vi "rscmwLS-lv2010_LTE_Signaling_example-1.0.0.vi"() -> ()   [LabVIEW 2010]
uses:
  <vilib>/Utility/error.llb/DialogType.ctl
panel:
  out "Error during execution?":bool
  out "State Indicator":T1(ring)
  out "RSRQ range":string
  out "RSRP range":string
  out "RSRQ":i32
  out "RSRP":i32
  out "error out":errorcluster
  in  "Set Type (Alternative Pattern)":i32(ring)=4 items=["Minimum Power", "Maximum Power", "Constant", "Single Pattern", "Closed Loop Target Power", "Different Pattern", "Continuous Pattern", "Alternative Pattern", "Relative Power Control"]
  in  "PUSCH Closed Loop Target Power (-20.0)":dbl=-20.0 caption="Power (-20.0)" format="%^.3e"
  in  "PUSCH Open Loop Nominal Power (-20.0)":dbl=-20.0 caption="Open Loop Nominal Power (-20.0)" format="%^.3e"
  in  "RS EPRE (-85.0)":dbl=-85.0 format="%^.3e"
  in  "Operating Band (Band 7)":i32(ring)=7 items=["User Defined"=0, "Band 1"=1, "Band 2"=2, "Band 3"=3, "Band 4"=4, "Band 5"=5, "Band 6"=6, "Band 7"=7, "Band 8"=8, "Band 9"=9, "Band 10"=10, "Band 11"=11, "Band 12"=12, "Band 13"=13, "Band 14"=14, "Band 15"=15, "Band 16"=16, "Band 17"=17, "Band 18"=18, "Band 19"=19, "Band 20"=20, "Band 21"=21, "Band 22"=22, "Band 23"=23, "Band 24"=24, "Band 25"=25, "Band 26"=26, "Band 27"=27, "Band 28"=28, "Band 29"=29, "Band 30"=30, "Band 31"=31, "Band 32"=32, "Band 33"=33, "Band 34"=34, "Band 35"=35, "Band 36"=36, "Band 37"=37, "Band 38"=38, "Band 39"=39, "Band 40"=40, "Band 41"=41, "Band 42"=42, "Band 43"=43, "Band 44"=44, "Band 252"=252, "Band 255"=255]
  in  "External Output Attenuation (0.0)":dbl caption="External Attenuation (0.0)" format="%^_3e"
  in  "External Input Attenuation (0.0)":dbl caption="External Attenuation (0.0)" format="%^_3e"
  in  "Duplex Mode (FDD)":i32(ring) items=["FDD", "TDD"]
  in  "RF Output Connector (RF 1 COM)":i32(ring)=1 items=["RF 1 OUT", "RF 1 COM", "RF 2 COM", "RF 3 OUT", "RF 3 COM", "RF 4 COM", "Virtual RF A", "Virtual RF B", "Virtual RF OUT"]
  in  "RF Output Converter (TX 1)":i32(ring) items=["TX 1", "TX 2", "TX 3", "TX 4"]
  in  "RF Input Converter (RX 1)":i32(ring) items=["RX 1", "RX 2", "RX 3", "RX 4"]
  in  "RF Input Connector (RF 1 COM)":i32(ring) items=["RF 1 COM", "RF 2 COM", "RF 3 COM", "RF 4 COM", "Virtual RF COM A", "Virtual RF COM B"]
  out "IP Address":string caption="IPv4 Address"
  out "IMSI":string
  out "IMEI":string
  in  "Instrument Descriptor (VISA resource name)":refnum<visa-resource-name>="TCPIP::CMW50050-156041::inst0::INSTR"
  # "Rohde & Schwarz CMW500 RF Tester\nLTE Signaling Example"
  # "Step 1: VISA resource name\nBefore running, change the Instrument Descriptor to fit your device:\nfor LAN: \"TCPIP::<ip_address>::<socket_number>::SOCKET\"\nfor VXI-11: \"TCPIP::<ip_address>::inst<i>::INSTR\"\nfor GPIB: \"GPIB::<address_number>::INSTR\""
  # "Step 3: Query UE information"
  # "Step 2: CMW LTE signaling settings\nBefore running, change the LTE signaling parameters to fit your UE's \nrequirements accordingly."
  # "Step 4: Read RSRP and RSRQ"
  # "Tested with R&S®CMW500 BASE FW 3.5.130 and R&S®CMW500 LTE UE FW 3.5.50\nBased on R&S®CMW500 LTE Signaling 3.5.400 (rscmwls) LabVIEW drivers\n\nDownloaded from: https://www.rohde-schwarz.com/driver/cmw500/\n\nChristian Wicke, Rohde & Schwarz International GmbH"
  # "State Maschine and LabVIEW Feedback"
  # "State Maschine Cases"
  # "as an example"
  # "as an example"
  # "Constant Settings"
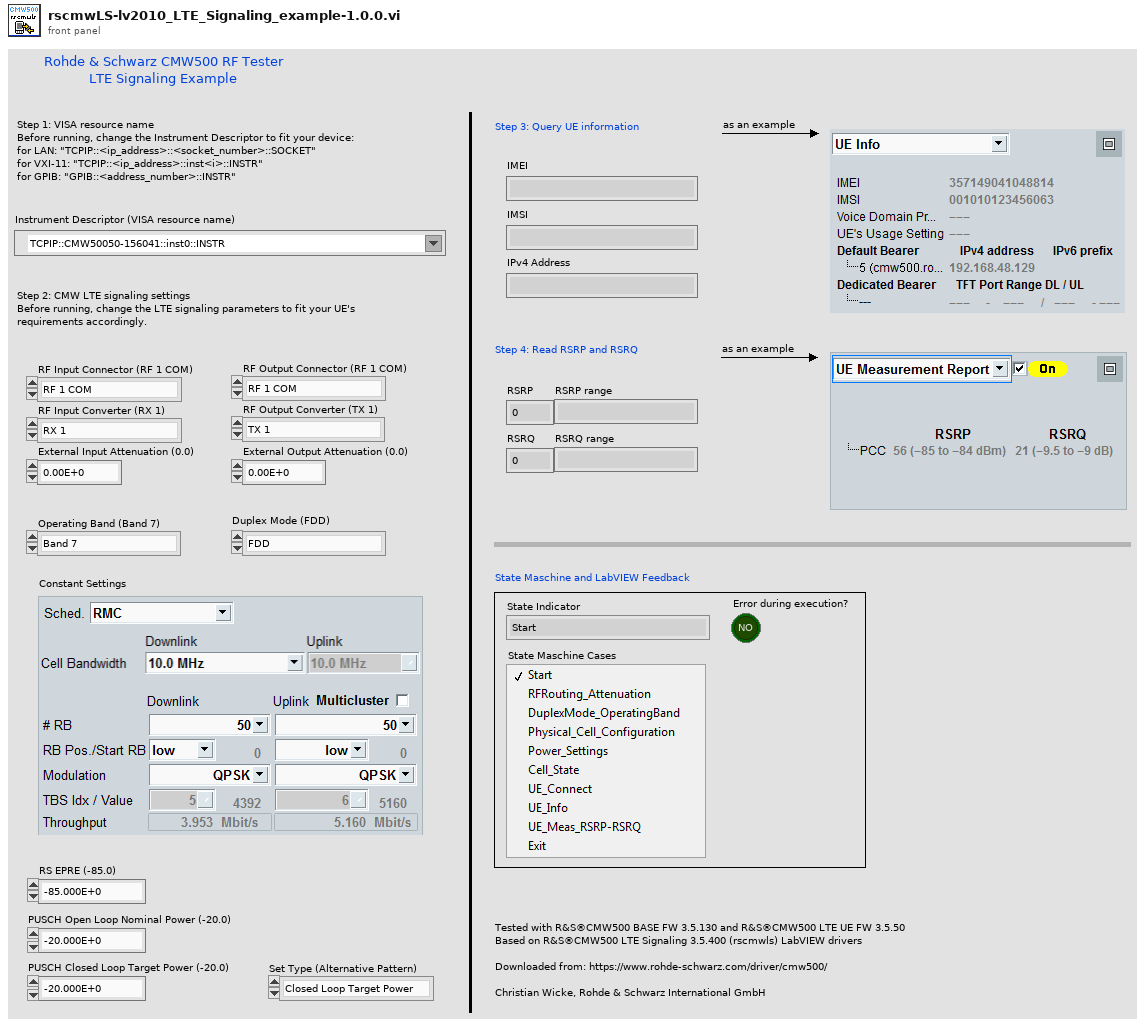
[diagram p1: front panel]
types:
  T1 = enum16{"Start", "RFRouting_Attenuation", "DuplexMode_OperatingBand", "Physical_Cell_Configuration", "Power_Settings", "Cell_State", "UE_Connect", "UE_Info", "UE_Meas_RSRP-RSRQ", "Exit"}
  T2 = typedef "DialogType.ctl" = u16
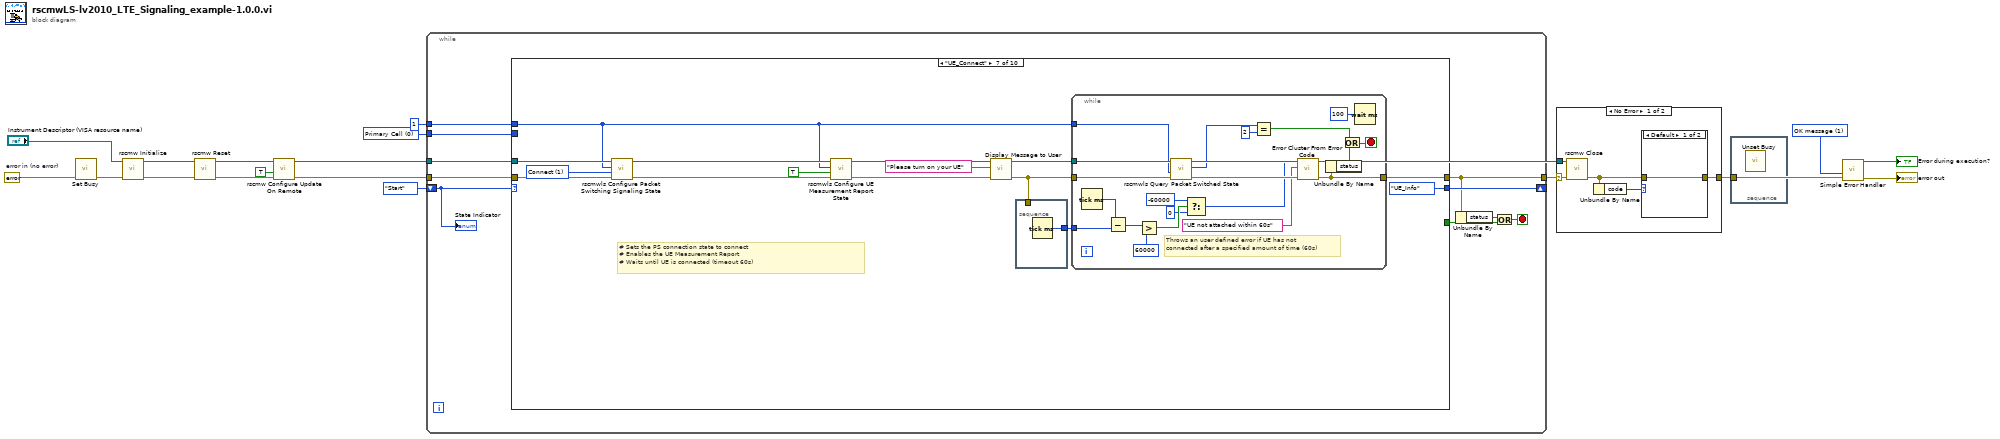
[diagram p0: block diagram]
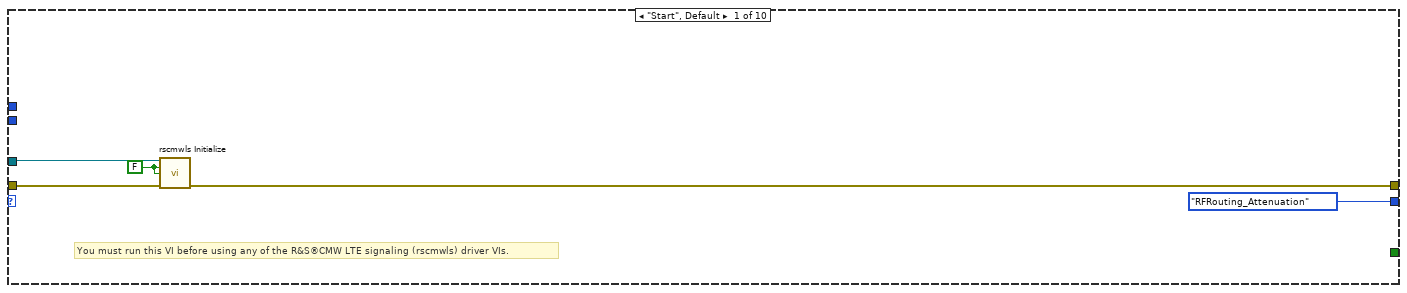
[diagram p4: hidden frame]
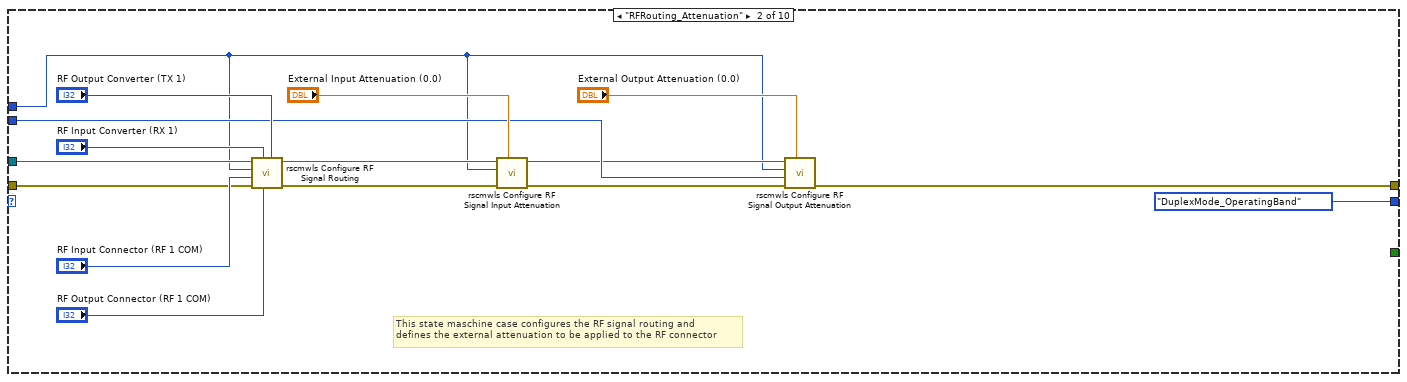
[diagram p5: hidden frame]
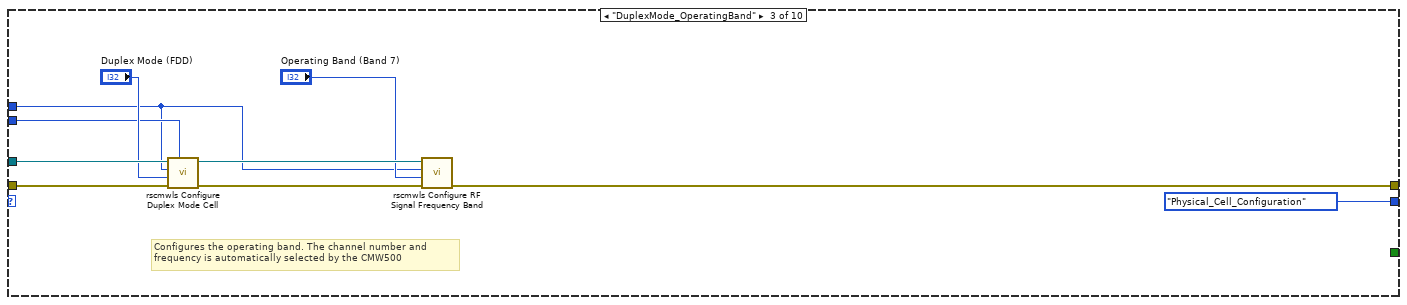
[diagram p6: hidden frame]
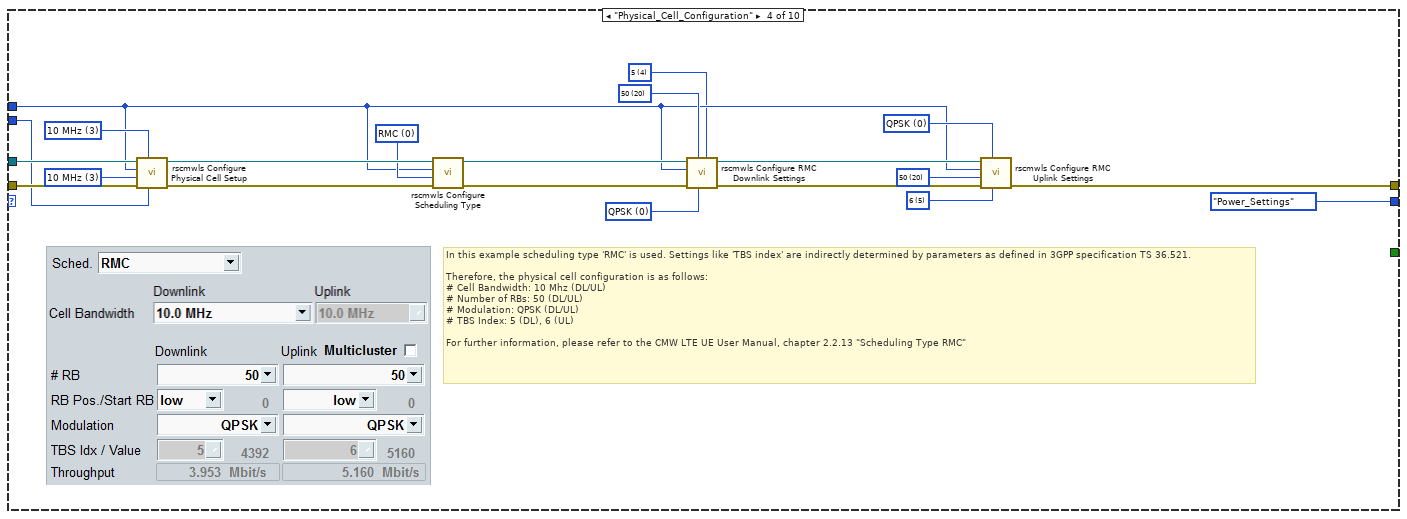
[diagram p7: hidden frame]
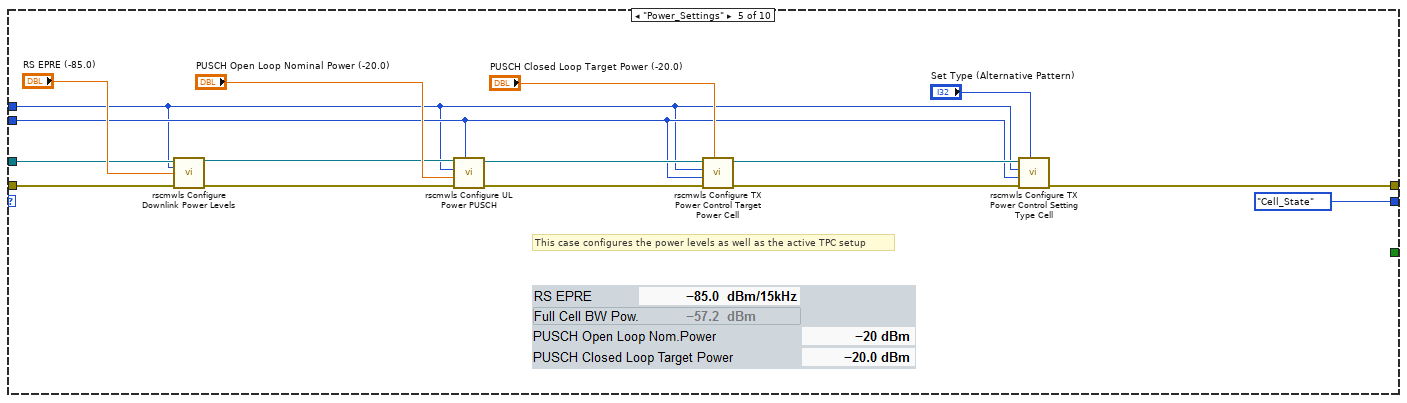
[diagram p8: hidden frame]
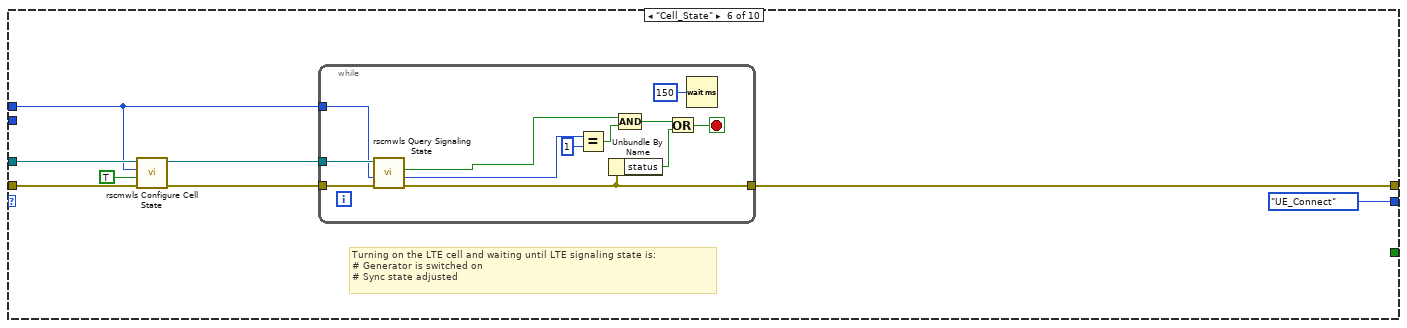
[diagram p9: hidden frame]
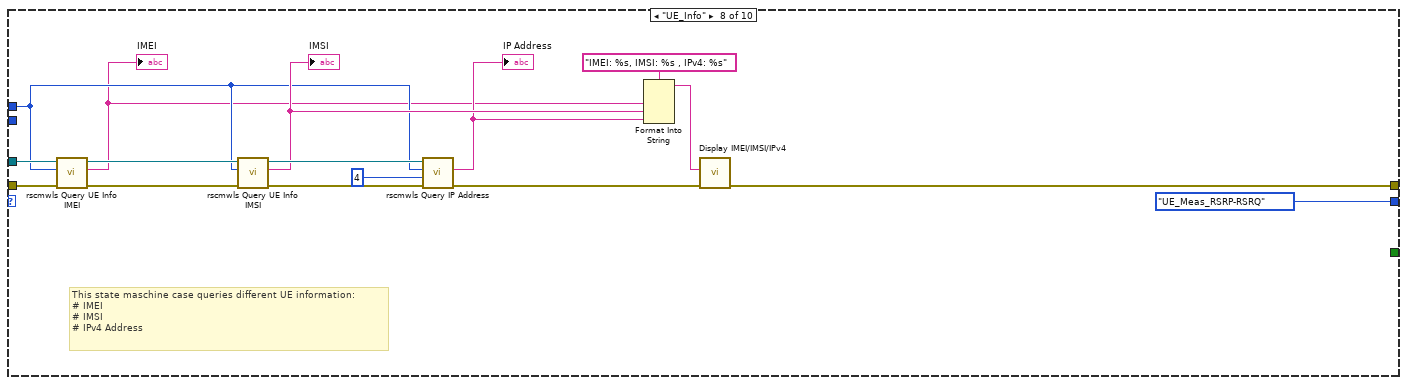
[diagram p10: hidden frame]
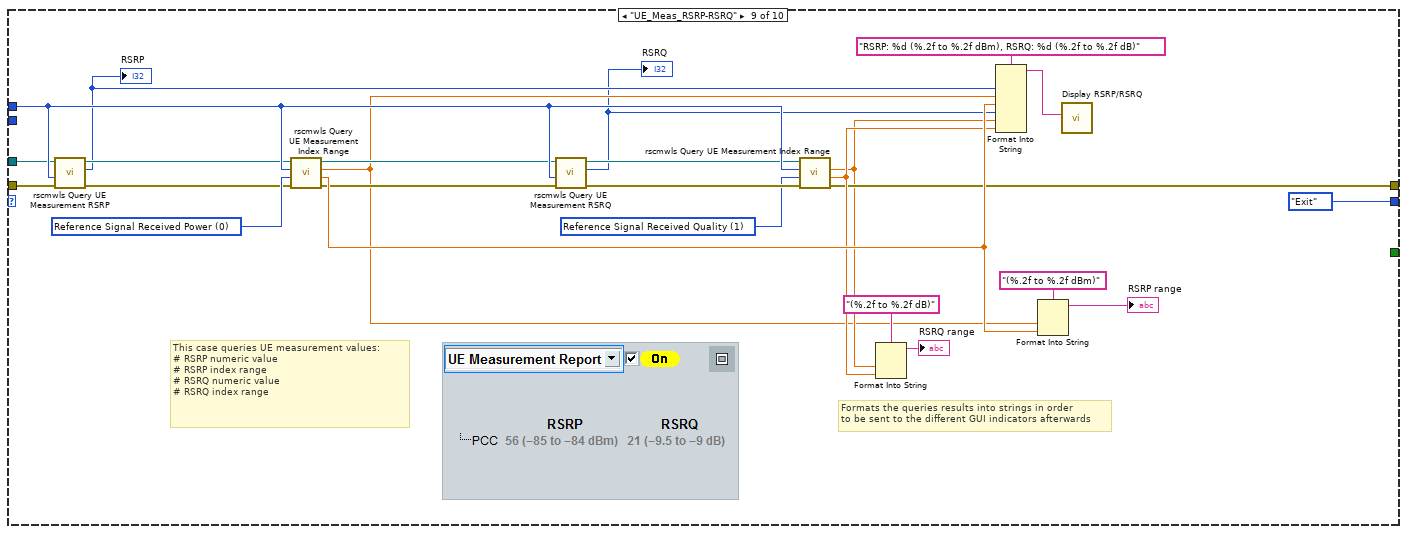
[diagram p11: hidden frame]
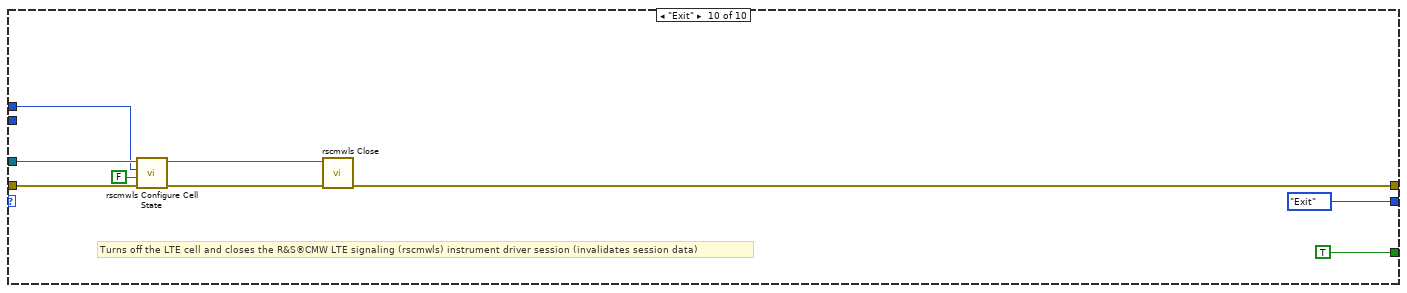
[diagram p12: hidden frame]
diagram:
  w5 = T2 1 items=["no dialog", "OK message", "continue or stop message", "OK message + warnings", "continue/stop + warnings"] ("type of dialog (OK msg:1)")
  w13 = 0 items=["Primary Cell", "Secondary Component Carrier 1", "Secondary Component Carrier 2", "Secondary Component Carrier 3"] ("Cell (Primary Cell)")
  w11 = errorcluster {"status"=FALSE, "code"=0, "source"=""}  # error in (no error)
  n1 = call <vilib>:"Set Busy.vi"("error in (no error)"=w11) -> ("error out"=w12:errorcluster)  [unwired: 9 in, 1 out]
  n2 = call <instrlib>:"rscmw Initialize.vi"("VISA resource name"="Instrument Descriptor (VISA resource name)", "error in (no error)"=w12) -> ("VISA resource name out"=w16:refnum<visa-resource-name>, "error out"=w17:errorcluster)  [unwired: 12 in]
  n3 = call <instrlib>:"rscmw Reset.vi"("VISA resource name"=w16, "error in (no error)"=w17) -> ("VISA resource name out"=w7:refnum<visa-resource-name>, "error out"=w8:errorcluster)  [unwired: 12 in]
  n4 = call <instrlib>:"rscmw Configure Update On Remote.vi"("error in (no error)"=w8, "Update (Off)"=TRUE, "VISA resource name"=w7) -> ("error out"=w6:errorcluster, "VISA resource name out"=w4:refnum<visa-resource-name>)  [unwired: 7 in]
  n5 = while {
    shift-right: [w22] -> _
    shift-left: T1."Start" -> [w23]
    tunnel: [w19] -> w3
    tunnel: w6 -> [w21]
    tunnel: w4 -> [w20]
    tunnel: 1 ("Instance (1)") -> [w28]
    tunnel: w13 -> [w27]
    stop <- w25 stop-if-true
    n6 = case shown="\"UE_Connect\"" w23 {
      tunnel: [w32 w44 w52 w67 w95 w98 w118 w158 w181 w193] -> w19
      tunnel: w21 -> [w31 w40 w58 w79 w90 w103 w129 w163 w180 w199]
      tunnel: w20 -> [w29 w39 w59 w80 w89 w104 w130 w162 w179 w200]
      tunnel: w28 -> [_ w34 w51 w65 w81 w99 w122 w155 w189 w197]
      tunnel: w27 -> [_ w42 w56 w60 w82 _ _ _ _ _]
      tunnel: [_ _ _ _ _ _ _ _ _ TRUE] -> w24
      tunnel: [T1."RFRouting_Attenuation" T1."DuplexMode_OperatingBand" T1."Physical_Cell_Configuration" T1."Power_Settings" T1."Cell_State" T1."UE_Connect" T1."UE_Info" T1."UE_Meas_RSRP-RSRQ" T1."Exit" T1."Exit"] -> w22
      frame "Start", Default {
        w33 = FALSE ("Reset (T: Reset)")
        # "You must run this VI before using any of the R&S®CMW LTE signaling (rscmwls) driver VIs."
        n7 = call <instrlib>:"rscmwls Initialize.vi"("VISA resource name"=w29, "ID Query (T: Check)"=w33, "Reset (T: Reset)"=w33, "error in (no error)"=w31) -> ("error out"=w32:errorcluster)  [unwired: 10 in, 1 out]
      }
      frame "RFRouting_Attenuation" {
        # "This state maschine case configures the RF signal routing and \ndefines the external attenuation to be applied to the RF connector"
        n8 = call <instrlib>:"rscmwls Configure RF Signal Routing.vi"("RF Output Converter (TX 1)"="RF Output Converter (TX 1)", "RF Output Connector (RF 1 COM)"="RF Output Connector (RF 1 COM)", "RF Input Converter (RX 1)"="RF Input Converter (RX 1)", "error in (no error)"=w40, "RF Input Connector (RF 1 COM)"="RF Input Connector (RF 1 COM)", "Instance (1)"=w34, "VISA resource name"=w39) -> ("error out"=w38:errorcluster, "VISA resource name out"=w37:refnum<visa-resource-name>)  [unwired: 3 in]
        n9 = call <instrlib>:"rscmwls Configure RF Signal Input Attenuation.vi"("External Attenuation (0.0)"="External Input Attenuation (0.0)", "error in (no error)"=w38, "Instance (1)"=w34, "VISA resource name"=w37) -> ("error out"=w36:errorcluster, "VISA resource name out"=w35:refnum<visa-resource-name>)  [unwired: 6 in]
        n10 = call <instrlib>:"rscmwls Configure RF Signal Output Attenuation.vi"("External Attenuation (0.0)"="External Output Attenuation (0.0)", "error in (no error)"=w36, "Cell (Primary Cell)"=w42, "Instance (1)"=w34, "VISA resource name"=w35) -> ("error out"=w44:errorcluster)  [unwired: 5 in, 1 out]
      }
      frame "DuplexMode_OperatingBand" {
        # "Configures the operating band. The channel number and \nfrequency is automatically selected by the CMW500"
        n11 = call <instrlib>:"rscmwls Configure Duplex Mode Cell.vi"("Cell (Primary Cell)"=w56, "error in (no error)"=w58, "Duplex Mode (FDD)"="Duplex Mode (FDD)", "Instance (1)"=w51, "VISA resource name"=w59) -> ("error out"=w55:errorcluster, "VISA resource name out"=w54:refnum<visa-resource-name>)  [unwired: 5 in]
        n12 = call <instrlib>:"rscmwls Configure RF Signal Frequency Band.vi"("error in (no error)"=w55, "Operating Band (Band 1)"="Operating Band (Band 7)", "Instance (1)"=w51, "VISA resource name"=w54) -> ("error out"=w52:errorcluster)  [unwired: 6 in, 1 out]
      }
      frame "Physical_Cell_Configuration" {
        w62 = 5 items=["Keep Compatible"=-2, "Zero"=-1, "1"=0, "2"=1, "3"=2, "4"=3, "5"=4, "6"=5, "11"=6, "12"=15, "13"=7, "14"=8, "18"=14, "19"=9, "21"=10, "23"=11, "24"=12, "25"=13] ("Transport Block Size Index (5)")
        w63 = 4 items=["Keep Compatible"=-2, "0"=-1, "1"=0, "2"=1, "3"=2, "4"=3, "5"=4, "6"=5, "7"=16, "11"=6, "12"=15, "13"=7, "14"=8, "17"=17, "18"=14, "19"=9, "21"=10, "22"=18, "23"=11, "24"=12, "25"=13] ("Transport Block Size Index (5)")
        w64 = 20 items=["Zero"=-1, "1"=0, "2"=1, "3"=2, "4"=3, "5"=4, "6"=5, "7"=30, "8"=6, "9"=24, "10"=7, "12"=8, "15"=9, "16"=10, "17"=26, "18"=11, "20"=12, "24"=13, "25"=14, "27"=15, "30"=16, "32"=27, "36"=17, "40"=18, "42"=31, "45"=28, "48"=19, "50"=20, "54"=25, "60"=29, "64"=32, "75"=21, "80"=22, "83"=35, "92"=33, "96"=34, "100"=23] ("Number Of RBs Uplink (50)")
        w66 = 0 items=["QPSK", "16-QAM", "64-QAM"] ("UL Modulation Type (QPSK)")
        w69 = 0 items=["QPSK", "16-QAM", "64-QAM"] ("DL Modulation Type (QPSK)")
        w68 = 20 items=["Zero"=-1, "1"=0, "2"=1, "3"=2, "4"=3, "5"=4, "6"=5, "7"=30, "8"=6, "9"=24, "10"=7, "12"=8, "15"=9, "16"=10, "17"=26, "18"=11, "20"=12, "24"=13, "25"=14, "27"=15, "30"=16, "32"=27, "36"=17, "40"=18, "42"=31, "45"=28, "48"=19, "50"=20, "54"=25, "60"=29, "64"=32, "75"=21, "80"=22, "83"=35, "92"=33, "96"=34, "100"=23] ("Number Of RBs Downlink (50)")
        w72 = 3 items=["1.4 MHz", "3 MHz", "5 MHz", "10 MHz", "15 MHz", "20 MHz"] ("DL Cell Bandwidth (10 MHz)")
        w71 = 3 items=["1.4 MHz", "3 MHz", "5 MHz", "10 MHz", "15 MHz", "20 MHz"] ("UL Cell Bandwidth (10 MHz)")
        w70 = 0 items=["RMC", "User defined channel", "User defined TTI Based", "CQI TTI Based", "CQI Follow WB", "CQI Follow WB PMI", "CQI Follow WB CQI-PMI-RI", "CQI Follow WB CQI-RI", "Semi-persistent scheduling", "CQI follow wideband PMI-RI"] ("Scheduling Type (RMC)")
        # "In this example scheduling type 'RMC' is used. Settings like 'TBS index' are indirectly determined by parameters as defined in 3GPP specification TS 36.521.\n\nTherefore, the physical cell configuration is as follows:\n# Cell Bandwidth: 10 Mhz (DL/UL)\n# Number of RBs: 50 (DL/UL)\n# Modulation: QPSK (DL/UL)\n# TBS Index: 5 (DL), 6 (UL)\n\nFor further information, please refer to the CMW LTE UE User Manual, chapter 2.2.13 \"Scheduling Type RMC\""
        n13 = call <instrlib>:"rscmwls Configure Physical Cell Setup.vi"("Physical Cell ID (0)"=w60, "UL Cell Bandwidth (10 MHz)"=w71, "error in (no error)"=w79, "DL Cell Bandwidth (10 MHz)"=w72, "Instance (1)"=w65, "VISA resource name"=w80) -> ("error out"=w78:errorcluster, "VISA resource name out"=w77:refnum<visa-resource-name>)  [unwired: 4 in]
        n14 = call <instrlib>:"rscmwls Configure Scheduling Type.vi"("error in (no error)"=w78, "Scheduling Type (RMC)"=w70, "Instance (1)"=w65, "VISA resource name"=w77) -> ("error out"=w76:errorcluster, "VISA resource name out"=w75:refnum<visa-resource-name>)  [unwired: 6 in]
        n15 = call <instrlib>:"rscmwls Configure RMC Downlink Settings.vi"("Transport Block Size Index (5)"=w63, "Modulation Type (QPSK)"=w69, "Number Of Resource Blocks (50)"=w68, "error in (no error)"=w76, "Instance (1)"=w65, "VISA resource name"=w75) -> ("error out"=w74:errorcluster, "VISA resource name out"=w73:refnum<visa-resource-name>)  [unwired: 4 in]
        n16 = call <instrlib>:"rscmwls Configure RMC Uplink Settings.vi"("Transport Block Size Index (5)"=w62, "Modulation Type (QPSK)"=w66, "error in (no error)"=w74, "Number Of Resource Blocks (50)"=w64, "Instance (1)"=w65, "VISA resource name"=w73) -> ("error out"=w67:errorcluster)  [unwired: 4 in, 1 out]
      }
      frame "Power_Settings" {
        # "This case configures the power levels as well as the active TPC setup"
        n17 = call <instrlib>:"rscmwls Configure Downlink Power Levels.vi"("VISA resource name"=w89, "Instance (1)"=w81, "RS EPRE (-85.0)"="RS EPRE (-85.0)", "error in (no error)"=w90) -> ("VISA resource name out"=w87:refnum<visa-resource-name>, "error out"=w88:errorcluster)  [unwired: 10 in]
        n18 = call <instrlib>:"rscmwls Configure UL Power PUSCH.vi"("Cell (Primary Cell)"=w82, "error in (no error)"=w88, "Open Loop Nominal Power (-20.0)"="PUSCH Open Loop Nominal Power (-20.0)", "Instance (1)"=w81, "VISA resource name"=w87) -> ("error out"=w86:errorcluster, "VISA resource name out"=w85:refnum<visa-resource-name>)  [unwired: 5 in]
        n19 = call <instrlib>:"rscmwls Configure TX Power Control Target Power Cell.vi"("Power (-20.0)"="PUSCH Closed Loop Target Power (-20.0)", "error in (no error)"=w86, "Cell (Primary Cell)"=w82, "Instance (1)"=w81, "VISA resource name"=w85) -> ("error out"=w84:errorcluster, "VISA resource name out"=w83:refnum<visa-resource-name>)  [unwired: 5 in]
        n20 = call <instrlib>:"rscmwls Configure TX Power Control Setting Type Cell.vi"("Set Type (Closed Loop Target Power)"="Set Type (Alternative Pattern)", "error in (no error)"=w84, "Cell (Primary Cell)"=w82, "Instance (1)"=w81, "VISA resource name"=w83) -> ("error out"=w95:errorcluster)  [unwired: 5 in, 1 out]
      }
      frame "Cell_State" {
        # "Turning on the LTE cell and waiting until LTE signaling state is:\n# Generator is switched on\n# Sync state adjusted"
        n21 = call <instrlib>:"rscmwls Configure Cell State.vi"("error in (no error)"=w103, "Cell State (Off)"=TRUE, "Instance (1)"=w99, "VISA resource name"=w104) -> ("error out"=w101:errorcluster, "VISA resource name out"=w100:refnum<visa-resource-name>)  [unwired: 6 in]
        n22 = while {
          tunnel: [w106] -> w98
          tunnel: w101 -> [w111]
          tunnel: w100 -> [w110]
          tunnel: w99 -> [w109]
          stop <- w116 stop-if-true
          n23 = call <instrlib>:"rscmwls Query Signaling State.vi"("error in (no error)"=w111, "Instance (1)"=w109, "VISA resource name"=w110) -> ("error out"=w106:errorcluster, "Sync State"=w113:i32, "Main State"=w105:bool)  [unwired: 5 in, 1 out]
          n24 = Equal?(x=w113, y=1) -> (x = y?=w108:bool)
          n25 = Unbundle By Name(w106) -> ("status"=w115:bool)
          n26 = Compound Arithmetic op=AND(w105, w108) -> (w112:bool)
          n27 = Or(x=w112, y=w115) -> (x .or. y?=w116:bool)
          n28 = Wait (ms)(milliseconds to wait=u32 150) -> ()  [unwired: 1 out]
        }
      }
      frame "UE_Connect" {
        w120 = 1 items=["Disconnect", "Connect", "Send SMS", "Detach", "Handover"] ("Action (Connect)")
        # "# Sets the PS connection state to connect\n# Enables the UE Measurement Report\n# Waits until UE is connected (timeout 60s)"
        n29 = call <instrlib>:"rscmwls Configure Packet Switching Signaling State.vi"("error in (no error)"=w129, "Action (Connect)"=w120, "Instance (1)"=w122, "VISA resource name"=w130) -> ("error out"=w127:errorcluster, "VISA resource name out"=w128:refnum<visa-resource-name>)  [unwired: 6 in]
        n30 = call <instrlib>:"rscmwls Configure UE Measurement Report State.vi"("error in (no error)"=w127, "Enable (Off)"=TRUE, "Instance (1)"=w122, "VISA resource name"=w128) -> ("error out"=w125:errorcluster, "VISA resource name out"=w123:refnum<visa-resource-name>)  [unwired: 6 in]
        n31 = call "Display Message to User"("error in (no error)"=w125, "Message"="Please turn on your UE") -> ("error out"=w117:errorcluster)  [unwired: 8 in, 1 out]
        n32 = stacked-sequence {
          tunnel: [w131] -> w119
          tunnel: w117 -> [_]
          frame #0 {
            n33 = Tick Count (ms)() -> (millisecond timer value=w131:u32)
          }
        }
        n34 = while {
          tunnel: w117 -> [w148]
          tunnel: w123 -> [w145]
          tunnel: w122 -> [w144]
          tunnel: w119 -> [w142]
          tunnel: [w132] -> w118
          stop <- w146 stop-if-true
          # "Throws an user defined error if UE has not\nconnected after a specified amount of time (60s)"
          n35 = Tick Count (ms)() -> (millisecond timer value=w143:u32)
          n36 = Subtract(x=w143, y=w142) -> (x-y=w138:u32)
          n37 = Greater?(x=w138, y=u32 60000) -> (0:w136:bool)
          n38 = call <instrlib>:"rscmwls Query Packet Switched State.vi"("error in (no error)"=w148, "Instance (1)"=w144, "VISA resource name"=w145) -> ("error out"=w141:errorcluster, "Connection State"=w151:i32)  [unwired: 6 in, 1 out]
          n39 = Select(t=-60000 ("error code (0)"), s=w136, f=0) -> (s? t:f=w139:i32)
          n40 = Equal?(x=w151, y=2) -> (x = y?=w140:bool)
          n41 = call <vilib>:"Error Cluster From Error Code.vi"("error in (no error)"=w141, "error message (\"\")"="UE not attached within 60s" ("error message (\"\")"), "error code (0)"=w139) -> ("error out"=w132:errorcluster)  [unwired: 6 in]
          n42 = Unbundle By Name(w132) -> ("status"=w147:bool)
          n43 = Or(x=w140, y=w147) -> (x .or. y?=w146:bool)
          n44 = Wait (ms)(milliseconds to wait=u32 100) -> ()  [unwired: 1 out]
        }
      }
      frame "UE_Info" {
        # "This state maschine case queries different UE information:\n# IMEI\n# IMSI\n# IPv4 Address"
        n45 = call <instrlib>:"rscmwls Query UE Info IMEI.vi"("error in (no error)"=w163, "Instance (1)"=w155, "VISA resource name"=w162) -> ("error out"=w164:errorcluster, "IMEI"=w153:string, "VISA resource name out"=w165:refnum<visa-resource-name>)  [unwired: 6 in]
        "IMEI" <- w153
        n46 = call <instrlib>:"rscmwls Query UE Info IMSI.vi"("error in (no error)"=w164, "Instance (1)"=w155, "VISA resource name"=w165) -> ("error out"=w166:errorcluster, "IMSI"=w159:string, "VISA resource name out"=w167:refnum<visa-resource-name>)  [unwired: 6 in]
        "IMSI" <- w159
        n47 = call <instrlib>:"rscmwls Query IP Address.vi"("error in (no error)"=w166, "IP Version (4)"=4, "Instance (1)"=w155, "VISA resource name"=w167) -> ("error out"=w152:errorcluster, "IP Address"=w154:string)  [unwired: 5 in, 1 out]
        "IP Address" <- w154
        n48 = Format Into String(format string="IMEI: %s, IMSI: %s , IPv4: %s", w153, w159, w154) -> (resulting string=w157:string)  [unwired: 2 in, 1 out]
        n49 = call "Display IMEI/IMSI/IPv4"("error in (no error)"=w152, "Message"=w157) -> ("error out"=w158:errorcluster)  [unwired: 8 in, 1 out]
      }
      frame "UE_Meas_RSRP-RSRQ" {
        w170 = 1 items=["Reference Signal Received Power", "Reference Signal Received Quality"] ("Report Type (Reference Signal Received Power)")
        w190 = 0 items=["Reference Signal Received Power", "Reference Signal Received Quality"] ("Report Type (Reference Signal Received Power)")
        # "Formats the queries results into strings in order\nto be sent to the different GUI indicators afterwards"
        # "This case queries UE measurement values:\n# RSRP numeric value\n# RSRP index range\n# RSRQ numeric value\n# RSRQ index range"
        n50 = call <instrlib>:"rscmwls Query UE Measurement RSRP.vi"("error in (no error)"=w180, "Instance (1)"=w189, "VISA resource name"=w179) -> ("error out"=w178:errorcluster, "RSRP"=w172:i32, "VISA resource name out"=w177:refnum<visa-resource-name>)  [unwired: 6 in]
        "RSRP" <- w172
        n51 = call <instrlib>:"rscmwls Query UE Measurement Index Range.vi"("error in (no error)"=w178, "Report Type (Reference Signal Received Power)"=w190, "Instance (1)"=w189, "VISA resource name"=w177) -> ("error out"=w176:errorcluster, "Upper"=w186:dbl, "Lower"=w169:dbl, "VISA resource name out"=w175:refnum<visa-resource-name>)  [unwired: 4 in]
        n52 = call <instrlib>:"rscmwls Query UE Measurement RSRQ.vi"("error in (no error)"=w176, "Instance (1)"=w189, "VISA resource name"=w175) -> ("error out"=w174:errorcluster, "RSRQ"=w168:i32, "VISA resource name out"=w173:refnum<visa-resource-name>)  [unwired: 6 in]
        "RSRQ" <- w168
        n53 = call <instrlib>:"rscmwls Query UE Measurement Index Range.vi"("error in (no error)"=w174, "Report Type (Reference Signal Received Power)"=w170, "Instance (1)"=w189, "VISA resource name"=w173) -> ("error out"=w181:errorcluster, "Upper"=w182:dbl, "Lower"=w171:dbl)  [unwired: 4 in, 1 out]
        n54 = Format Into String(format string="(%.2f to %.2f dB)" ("regular expression"), w171, w182) -> (resulting string=→"RSRQ range":string)  [unwired: 2 in, 1 out]
        n55 = Format Into String(format string="RSRP: %d (%.2f to %.2f dBm), RSRQ: %d (%.2f to %.2f dB)", w172, w169, w186, w168, w171, w182) -> (resulting string=w188:string)  [unwired: 2 in, 1 out]
        n56 = Format Into String(format string="(%.2f to %.2f dBm)" ("regular expression"), w169, w186) -> (resulting string=→"RSRP range":string)  [unwired: 2 in, 1 out]
        n57 = call "Display RSRP/RSRQ"("Message"=w188) -> ()  [unwired: 9 in, 2 out]
      }
      frame "Exit" {
        # "Turns off the LTE cell and closes the R&S®CMW LTE signaling (rscmwls) instrument driver session (invalidates session data)"
        n58 = call <instrlib>:"rscmwls Configure Cell State.vi"("error in (no error)"=w199, "Cell State (Off)"=FALSE, "Instance (1)"=w197, "VISA resource name"=w200) -> ("error out"=w195:errorcluster, "VISA resource name out"=w194:refnum<visa-resource-name>)  [unwired: 6 in]
        n59 = call <instrlib>:"rscmwls Close.vi"("error in (no error)"=w195, "VISA resource name"=w194) -> ("error out"=w193:errorcluster)  [unwired: 9 in]
      }
    }
    n60 = Unbundle By Name(w19) -> ("status"=w26:bool)
    n61 = Or(x=w26, y=w24) -> (x .or. y?=w25:bool)
    "State Indicator" <- w23
  }
  n62 = case shown="No Error" w3 {
    selector: w3 -> [w202 w208]
    tunnel: [w206 w208] -> w2
    tunnel: w4 -> [w203 _]
    frame No Error {
      n63 = call <instrlib>:"rscmw Close.vi"("error in (no error)"=w202, "VISA resource name"=w203) -> ("error out"=w205:errorcluster)  [unwired: 9 in]
      n64 = Unbundle By Name(w205) -> ("code"=w204:i32)
      n65 = case shown="Default" w204 {
        tunnel: [w207 _] -> w206
        tunnel: w205 -> [w207 _]
        frame Default {
        }
        frame 1073676418 {
        }
      }
    }
    frame Error {
    }
  }
  n66 = stacked-sequence {
    tunnel: w2 -> [_]
    frame #0 {
      n67 = call <vilib>:"Unset Busy.vi"() -> ()  [unwired: 11 in, 1 out]
    }
  }
  n68 = call <vilib>:"Simple Error Handler.vi"("type of dialog (OK msg:1)"=w5, "error in (no error)"=w2) -> ("error?"=→"Error during execution?":bool, "error out"=→"error out":errorcluster)  [unwired: 3 in, 3 out]
